vi "initEMCY.vi"(8 "error in (no error)":errorcluster, 10 "interface object in":refnum<k20>, 11 "MotorController in":refnum<class "MotorController.lvclass">) -> (0 "error out":errorcluster, 1 "emergency object out":refnum<k20>, 2 "interface object out":refnum<k20>, 3 "MotorController out":refnum<class "MotorController.lvclass">)   [LabVIEW 2017, in "MotorController.lvclass"]
uses:
  MotorController.lvclass
  MotorController.lvclass/MotorController.ctl
  <vilib>/CANopenLib/CANOPEN.llb/CANopen Emergency Create.vi
  <vilib>/CANopenLib/CANOPEN.llb/CANopen Emergency Start.vi
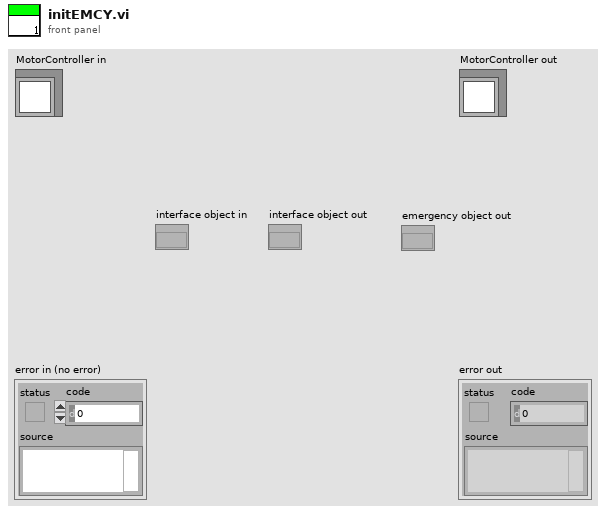
[diagram p1: front panel]
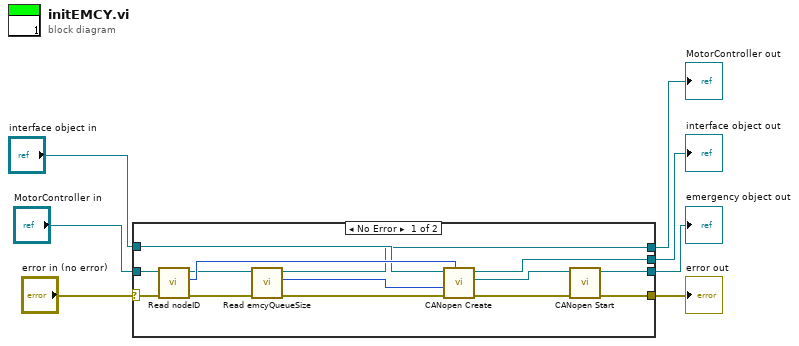
[diagram p0: block diagram]
diagram:
  n1 = case shown="No Error" "error in (no error)" {
    selector: "error in (no error)" -> [w13 w24]
    tunnel: [w10 w24] -> w6
    tunnel: [w8 w23] -> w4
    tunnel: "MotorController in" -> [w14 w23]
    tunnel: "interface object in" -> [w12 w22]
    tunnel: [w11 w22] -> w2
    tunnel: [w9 _] -> w1
    frame No Error {
      n2 = call "Read nodeID.vi"("error in (no error)"=w13, "MotorController in"=w14) -> ("error out"=w19:errorcluster, "nodeID"=w21:u8, "MotorController out"=w20:refnum<class "MotorController.lvclass">)  [unwired: 7 in]
      n3 = call "Read emcyQueueSize.vi"("error in (no error)"=w19, "MotorController in"=w20) -> ("error out"=w17:errorcluster, "emcyQueueSize"=w18:u16, "MotorController out"=w8:refnum<class "MotorController.lvclass">)  [unwired: 7 in]
      n4 = call-poly <vilib>:"CANopen Create.vi"("node-ID"=w21, "error in (no error)"=w17, "buffer size (0)"=w18, "interface object in"=w12) -> ("error out"=w15:errorcluster, "emergency object out"=w16:refnum<k20>, "interface object out"=w11:refnum<k20>)  [unwired: 5 in]
      n5 = call-poly <vilib>:"CANopen Start.vi"("error in (no error)"=w15, "emergency object in"=w16) -> ("error out"=w10:errorcluster, "emergency object out"=w9:refnum<k20>)  [unwired: 8 in]
    }
    frame Error {
    }
  }
  "error out" <- w6
  "MotorController out" <- w4
  "interface object out" <- w2
  "emergency object out" <- w1
